vi "Set Service Name.vi"(8 "error in (no error)":errorcluster, 10 "Service name":string, 11 "NI_AB_API_RESTful in":refnum<class "NI_AB_API_RESTful.lvclass">) -> (0 "error out":errorcluster, 3 "NI_AB_API_RESTful out":refnum<class "NI_AB_API_RESTful.lvclass">)   [LabVIEW 2020, in "NI_AB_API_RESTful.lvclass"]
uses:
  <vilib>/AppBuilder/AB_API/RESTful/NI_AB_API_RESTful.lvclass
  <vilib>/AppBuilder/AB_API/RESTful/NI_AB_API_RESTful.lvclass/NI_AB_API_RESTful.ctl
  <vilib>/AppBuilder/AB_API/Build/NI_AB_API_Build.lvclass
  <resource>/Framework/Providers/Common/provcom_StringGlobals.vi
  <vilib>/AppBuilder/AB_Classes/RESTful/AB_RESTfulWebService.lvclass
  e:/builds/penguin/labview/branches/2020/dev/dist/vi.lib/AppBuilder/AB_API/Targetfile/NI_AB_API_Targetfile.lvclass
  e:/builds/penguin/labview/branches/2020/dev/dist/vi.lib/AppBuilder/AB_API/Build/NI_AB_API_Build.lvclass
  e:/builds/penguin/labview/branches/2020/dev/dist/vi.lib/AppBuilder/AB_API/RESTful/NI_AB_API_RESTful.lvclass
  e:/builds/penguin/labview/branches/2020/dev/dist/vi.lib/AppBuilder/AB_Classes/WebService/AB_WebService.lvclass
  e:/builds/penguin/labview/branches/2020/dev/dist/vi.lib/AppBuilder/AB_Classes/TargetFile/AB_Targetfile.lvclass
  e:/builds/penguin/labview/branches/2020/dev/dist/vi.lib/AppBuilder/AB_Classes/Build/AB_Build.lvclass
  e:/builds/penguin/labview/branches/2020/dev/dist/vi.lib/AppBuilder/AB_Classes/RESTful/AB_RESTfulWebService.lvclass
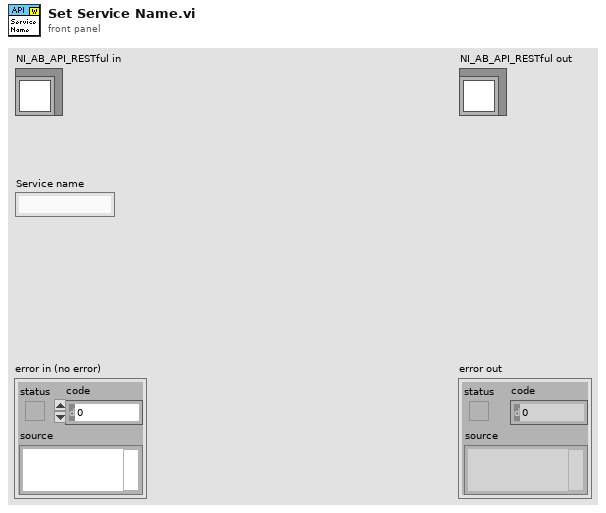
[diagram p1: front panel]
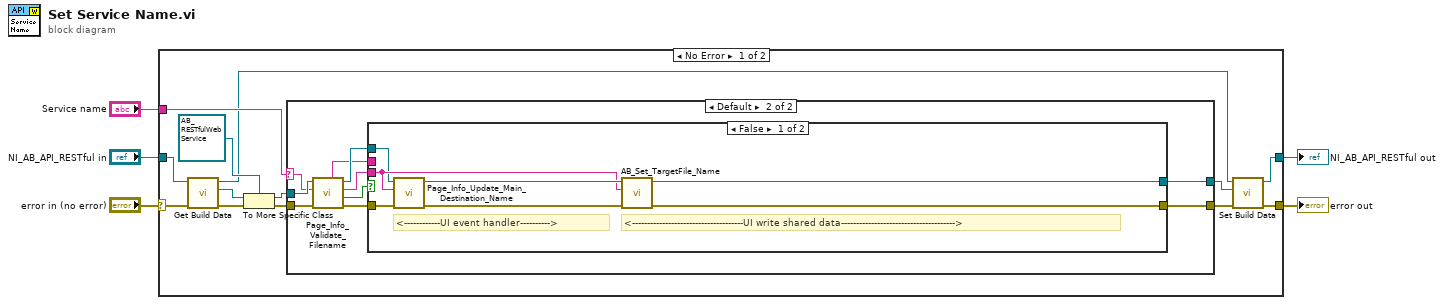
[diagram p0: block diagram]
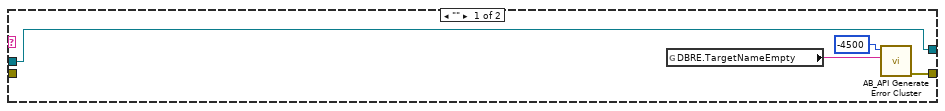
[diagram p2: hidden frame]
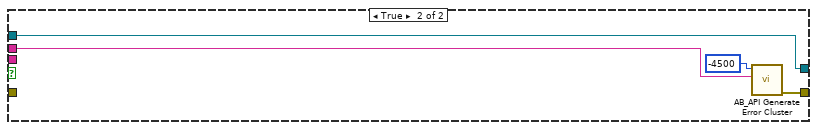
[diagram p3: hidden frame]
diagram:
  n1 = case shown="No Error" "error in (no error)" {
    selector: "error in (no error)" -> [w15 w45]
    tunnel: [w14 w45] -> w3
    tunnel: [w16 w44] -> w4
    tunnel: "NI_AB_API_RESTful in" -> [w17 w44]
    tunnel: "Service name" -> [w18 _]
    frame No Error {
      n2 = call <vilib>:"Get Build Data.vi"("error in (no error)"=w15, "NI_AB_API_Build in"=w17) -> ("error out"=w7:errorcluster, "AB_Build.lvclass"=w10:refnum<class "AB_Build.lvclass">, "NI_AB_API_Build out"=w9:refnum<class "NI_AB_API_RESTful.lvclass">)  [unwired: 7 in]
      n3 = To More Specific Class(target class=refnum<class "AB_RESTfulWebService.lvclass"> refnum ("AB_RESTfulWebService.lvclass"), reference=w10, error in=w7) -> (specific class reference=w8:refnum<class "AB_RESTfulWebService.lvclass">, error out=w6:errorcluster)
      n4 = case shown="Default" w18 {
        selector: w18 -> [_ w28]
        tunnel: [w20 w32] -> w13
        tunnel: w6 -> [_ w25]
        tunnel: w8 -> [w19 w30]
        tunnel: [w19 w31] -> w12
        frame "" {
          n5 = global read "provcom_StringGlobals.vi" "DBRE.TargetNameEmpty"() -> (w21:string)
          n6 = call <vilib>:"AB_API Generate Error Cluster.vi"("Additional Message"=w21, "Code"=-4500) -> ("error out"=w20:errorcluster)  [unwired: 2 in, 7 out]
        }
        frame Default {
          n7 = call-dynamic "Page_Info_Validate_Filename.vi"("error in (no error)"=w25, "Filename in"=w28, "AB_RESTfulWebService in"=w30) -> ("error out"=w24:errorcluster, "hasInvalidCharacters"=w26:bool, "Filename out"=w27:string, "AB_RESTfulWebService out"=w29:refnum<class "AB_RESTfulWebService.lvclass">, "message"=w23:string)  [unwired: 4 out]
          n8 = case shown="False" w26 {
            tunnel: [w38 w42] -> w32
            tunnel: w24 -> [w33 _]
            tunnel: w29 -> [w34 w41]
            tunnel: [w39 w41] -> w31
            tunnel: w27 -> [w35 _]
            tunnel: w23 -> [_ w40]
            frame False {
              # "<-------------------------------------UI write shared data-------------------------------------->"
              # "<------------UI event handler---------->"
              n9 = call-dynamic "Page_Info_Update_Main_Destination_Name.vi"("error in (no error)"=w33, "destination name"=w35, "AB_RESTfulWebService in"=w34) -> ("error out"=w36:errorcluster, "AB_RESTfulWebService out"=w37:refnum<class "AB_RESTfulWebService.lvclass">)  [unwired: 7 out]
              n10 = call <vilib>:"AB_Set_TargetFile_Name.vi"("error in (no error)"=w36, "Target filename"=w35, "TargetFile in"=w37) -> ("error out"=w38:errorcluster, "TargetFile out"=w39:refnum<class "AB_RESTfulWebService.lvclass">)  [unwired: 7 in]
            }
            frame True {
              n11 = call <vilib>:"AB_API Generate Error Cluster.vi"("Additional Message"=w40, "Code"=-4500) -> ("error out"=w42:errorcluster)  [unwired: 2 in, 7 out]
            }
          }
        }
      }
      n12 = call <vilib>:"Set Build Data.vi"("error in (no error)"=w13, "AB_Build.lvclass"=w12, "NI_AB_API_Build in"=w9) -> ("error out"=w14:errorcluster, "NI_AB_API_Build out"=w16:refnum<class "NI_AB_API_RESTful.lvclass">)  [unwired: 7 in]
    }
    frame Error {
    }
  }
  "error out" <- w3
  "NI_AB_API_RESTful out" <- w4
